vi "Truncate to 2 Digits.vi"(9 "Hours In":dbl, 10 "Minutes In":dbl, 11 "Sec In":dbl) -> (1 "Hours Out":dbl, 2 "Minutes Out":dbl, 3 "Sec Out":dbl)   [LabVIEW 2024, in "UIs Handler.lvlib"]
uses:
  UIs Handler.lvlib
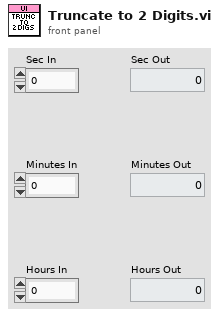
[diagram p1: front panel]
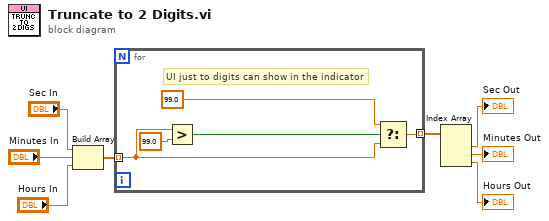
[diagram p0: block diagram]
diagram:
  n1 = Build Array("Sec In", "Minutes In", "Hours In") -> (w5:dbl[])
  n2 = for {
    tunnel: w5 -> [w9] mode=indexing
    tunnel: [w11] -> w4 mode=indexing
    # "UI just to digits can show in the indicator"
    n3 = Greater?(x=w9, y=99.0) -> (0:w12:bool)
    n4 = Select(t=99.0, s=w12, f=w9) -> (s? t:f=w11:dbl)
  }
  n5 = Index Array(array=w4) -> (element #1=→"Sec Out":dbl, element #2=→"Minutes Out":dbl, element #3=→"Hours Out":dbl)  [unwired: 3 in]
